vi "LabVIEW Data to Python String (CXT).vi"(8 "error in (no error)":errorcluster, 10 "LabVIEW Data":cxt) -> (0 "error out":errorcluster, 2 "Python String":string)   [LabVIEW 2020, in "jki_python_data_tools.lvlib"]
doc: "Writes a value associated with key in a specified section of the configuration data identified by refnum. If \"key\" input is not specified, the name of the variant object is used as the key.\n\nFor example a Boolean named \"Enable\" with a value of TRUE would correspond to the key-value pair:\n\nEnable=TRUE"
uses:
  jki_python_data_tools.lvlib
panel:
  # "Copyright © 2003-2009 JKI. All rights reserved.\n\nAuthor: Jim Kring [jim.kring@jameskring.com]\n\nThis library is provided \"AS IS\" ,WITHOUT WARRANTIES OR \nCONDITIONS OF ANY KIND, either express or implied.\n\nJames Kring, Inc. -- http://www.jameskring.com"
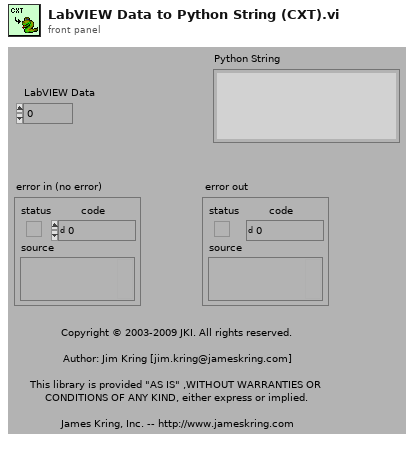
[diagram p1: front panel]
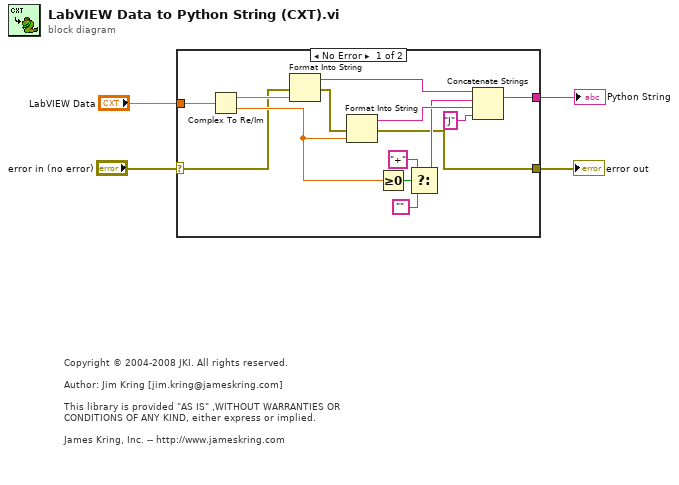
[diagram p0: block diagram]
diagram:
  # "Copyright © 2004-2008 JKI. All rights reserved.\n\nAuthor: Jim Kring [jim.kring@jameskring.com]\n\nThis library is provided \"AS IS\" ,WITHOUT WARRANTIES OR \nCONDITIONS OF ANY KIND, either express or implied.\n\nJames Kring, Inc. -- http://www.jameskring.com"
  n1 = case shown="No Error" "error in (no error)" {
    selector: "error in (no error)" -> [w5 w19]
    tunnel: "LabVIEW Data" -> [w8 _]
    tunnel: [w7 w19] -> w3
    tunnel: [w6 _] -> w2
    frame No Error {
      n2 = Complex To Re/Im(x + iy=w8) -> (x=w9:ext, y=w11:ext)
      n3 = Format Into String(error in=w5, w9) -> (resulting string=w17:string, error out=w10:errorcluster)  [unwired: 2 in]
      n4 = Format Into String(error in=w10, w11) -> (resulting string=w18:string, error out=w7:errorcluster)  [unwired: 2 in]
      n5 = Greater Or Equal To 0?(x=w11) -> (x >= 0?=w12:bool)
      n6 = Select(t="+" ("input 3"), s=w12, f="") -> (s? t:f=w16:string)
      n7 = Concatenate Strings(w17, w16, w18, "J" ("format string")) -> (w6:string)
    }
    frame Error {
    }
  }
  "error out" <- w3
  "Python String" <- w2
